vi "AMZ_S3_API_Create Grantee XML String (URI).vi"(4 "URI":string) -> (1 "Grantee":string)   [LabVIEW 2011, in "LV Interface for Amazon S3.lvlib"]
uses:
  LV Interface for Amazon S3.lvlib
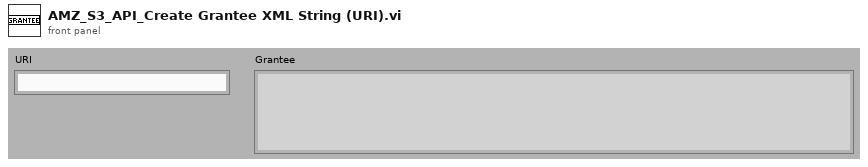
[diagram p1: front panel]
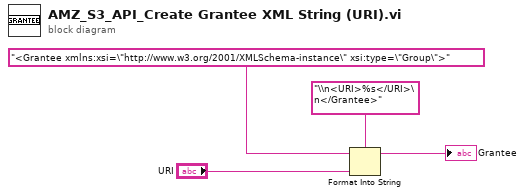
[diagram p0: block diagram]
diagram:
  n1 = Format Into String(format string="\\n<URI>%s</URI>\n</Grantee>", initial string="<Grantee xmlns:xsi=\"http://www.w3.org/2001/XMLSchema-instance\" xsi:type=\"Group\">", "URI") -> (resulting string=→"Grantee":string)  [unwired: 1 in, 1 out]
